vi "Get Gripper.vi"(8 "error in (no error)":errorcluster, 11 "KUKA youBot arm in":refnum<class "NI_Robotics_KUKA youBot Arm.lvclass">) -> (0 "error out":errorcluster, 2 "KUKA youBot gripper out":refnum<class "NI_Robotics_KUKA youBot Gripper.lvclass">, 3 "KUKA youBot arm out":refnum<class "NI_Robotics_KUKA youBot Arm.lvclass">)   [LabVIEW 2017, in "NI_Robotics_KUKA youBot Host.lvlib" / "NI_Robotics_KUKA youBot Arm.lvclass"]
doc: "Gets the KUKA youBot gripper instance from a KUKA youBot arm."
uses:
  <vilib>/robotics/KUKA youBot/Basic Device/Arm/NI_Robotics_KUKA youBot Arm.lvclass
  <vilib>/robotics/KUKA youBot/Basic Device/Gripper/NI_Robotics_KUKA youBot Gripper.lvclass
  <vilib>/robotics/KUKA youBot/Basic Device/Arm/NI_Robotics_KUKA youBot Arm.lvclass/NI_Robotics_KUKA youBot Arm.ctl
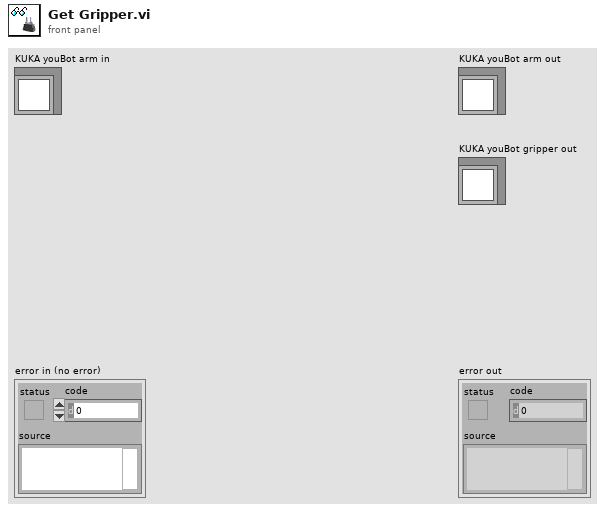
[diagram p1: front panel]
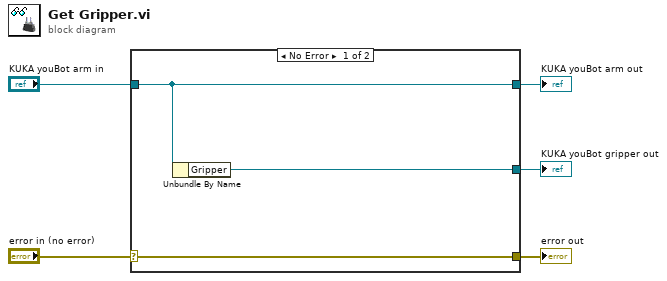
[diagram p0: block diagram]
diagram:
  n1 = case shown="No Error" "error in (no error)" {
    selector: "error in (no error)" -> [w8 w9]
    tunnel: [w8 w9] -> w4
    tunnel: [w7 w10] -> w2
    tunnel: "KUKA youBot arm in" -> [w7 w10]
    tunnel: [w6 _] -> w1
    frame No Error {
      n2 = Unbundle By Name(w7) -> ("Gripper"=w6:refnum<class "NI_Robotics_KUKA youBot Gripper.lvclass">)
    }
    frame Error {
    }
  }
  "error out" <- w4
  "KUKA youBot arm out" <- w2
  "KUKA youBot gripper out" <- w1
